vi "Log Reader.vi"() -> ()   [LabVIEW 2012]
uses:
  <vilib>/Utility/sysdir.llb/System Directory Type.ctl
  <vilib>/Utility/inputDevices.llb/closeKeyboard.vi
  <vilib>/Utility/inputDevices.llb/keyboardAcquire.vi
panel:
  in  "Cues":i32[](listbox)
  in  "stop":bool
  out "Total Length":u32
  out "Distance":string
  out "Current Pitch":dbl
  out "AutoTargetPitch":dbl
  out "AutoTargetRotation":dbl
  out "Auto Align":bool
  out "Fine Control Mode":bool
  out "SelectedGoalSubarray":dbl[](array[numeric])
  out "Vision Array":dbl[][](array[numeric])
  in  "-1 Frame":bool
  in  "+1 Frame":bool
  in  "Play Speed":dbl(slide)=1.0 step=0.25 scale=-5.0..5.0
  in  "Play/Pause":bool
  out "Image":T1(plugin-control)
  in  "Step":i32
  out "JS Buttons 3":T2
  out "Joystick 1":cluster{"X":dbl, "Y":dbl}[](graph)
  out "Joystick 2":cluster{"X":dbl, "Y":dbl}[](graph)
  out "JS Buttons 1":T2
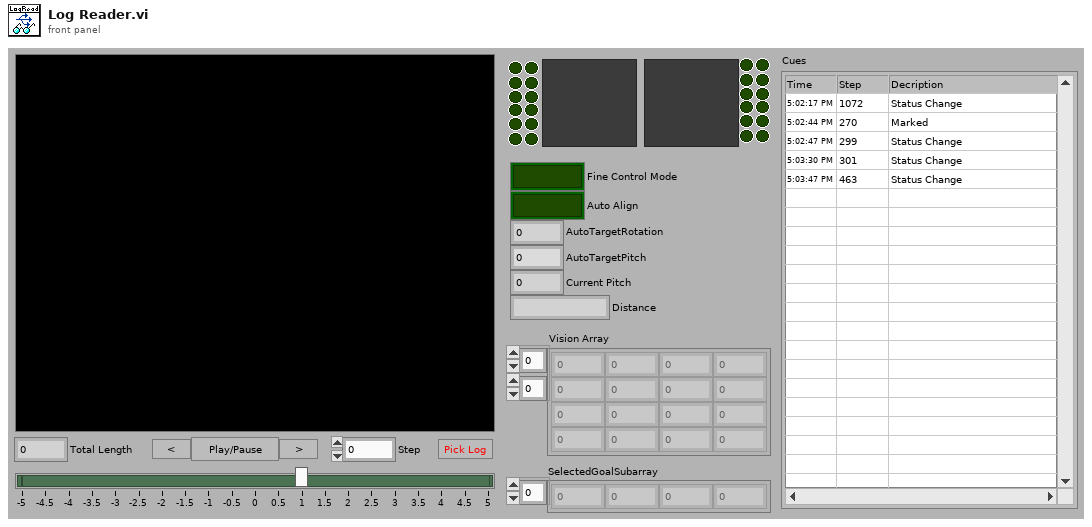
[diagram p1: front panel]
types:
  T1 = typedef "IMAQ Image.ctl" = refnum<image>
  T2 = cluster{bool, bool, bool, bool, bool, bool, bool, bool, bool, bool, bool, bool}
  T3 = cluster{"Joystick 1":cluster{"X":dbl, "Y":dbl}[], "JS Buttons 1":cluster{bool, bool, bool, bool, bool, bool, bool, bool, bool, bool, bool, bool}, "Joystick 2":cluster{"X":dbl, "Y":dbl}[], "JS Buttons 2":cluster{bool, bool, bool, bool, bool, bool, bool, bool, bool, bool, bool, bool}, "AutoTargetRotation":dbl, "AutoTargetPitch":dbl, "Fine Control Mode":bool, "Auto Align":bool, "Current Pitch":dbl, "Full Array":dbl[][], "SelectedGoalSubarray":dbl[], "Distance":string}
  T4 = enum16{"0", "1", "2", "3", "4", "5", "6", "7", "8", "9", "A", "B", "C", "D", "E", "F", "G", "H", "I", "J", "K", "L", "M", "N", "O", "P", "Q", "R", "S", "T", "U", "V", "W", "X", "Y", "Z", "F1", "F2", "F3", "F4", "F5", "F6", "F7", "F8", "F9", "F10", "F11", "F12", "F13", "F14", "F15", "ADD", "BACK", "BACKSLASH", "CAPITAL", "COMMA", "DECIMAL", "DELETE", "DIVIDE", "DOWN", "END", "EQUALS", "ESCAPE", "GRAVE (`)", "HOME", "INSERT", "LBRACKET", "LCONTROL", "LEFT", "L ALT", "LSHIFT", "LWIN", "MINUS", "MULTIPLY", "NEXT", "NUMLOCK", "NUMPAD_0", "NUMPAD_1", "NUMPAD_2", "NUMPAD_3", "NUMPAD_4", "NUMPAD_5", "NUMPAD_6", "NUMPAD_7", "NUMPAD_8", "NUMPAD_9", "PAUSE", "PERIOD", "PRIOR (PG UP)", "RBRACKET", "RCONTROL", "RETURN", "RIGHT", "R ALT", "RSHIFT", "RWIN", "SCROLL", "SEMICOLON", "SLASH", "SPACE", "SUBTRACT", "TAB", "UP", "ENTER (num pad)", "' (quote)"}
  T5 = typedef "System Directory Type.ctl" = i32
  T6 = typedef "Image Type" = u32
  T7 = typedef "AviRefnum.ctl" = refnum<k1>
  T8 = cluster{"Joystick 1":cluster{"X":dbl, "Y":dbl}[], "JS Buttons 1":cluster{bool, bool, bool, bool, bool, bool, bool, bool, bool, bool, bool, bool}, "Joystick 2":cluster{"X":dbl, "Y":dbl}[], "JS Buttons 2":cluster{bool, bool, bool, bool, bool, bool, bool, bool, bool, bool, bool, bool}, "AutoTargetRotation":dbl, "AutoTargetPitch":dbl, "Fine Control Mode":bool, "Auto Align":bool, "Current Pitch":dbl, "Full Array":dbl[][], "SelectedGoalSubarray":dbl[], "Distance":string}[]
  T9 = enum16{"0", "1", "2", "3", "4", "5", "6", "7", "8", "9", "A", "B", "C", "D", "E", "F", "G", "H", "I", "J", "K", "L", "M", "N", "O", "P", "Q", "R", "S", "T", "U", "V", "W", "X", "Y", "Z", "F1", "F2", "F3", "F4", "F5", "F6", "F7", "F8", "F9", "F10", "F11", "F12", "F13", "F14", "F15", "ADD", "BACK", "BACKSLASH", "CAPITAL", "COMMA", "DECIMAL", "DELETE", "DIVIDE", "DOWN", "END", "EQUALS", "ESCAPE", "GRAVE (`)", "HOME", "INSERT", "LBRACKET", "LCONTROL", "LEFT", "L ALT", "LSHIFT", "LWIN", "MINUS", "MULTIPLY", "NEXT", "NUMLOCK", "NUMPAD_0", "NUMPAD_1", "NUMPAD_2", "NUMPAD_3", "NUMPAD_4", "NUMPAD_5", "NUMPAD_6", "NUMPAD_7", "NUMPAD_8", "NUMPAD_9", "PAUSE", "PERIOD", "PRIOR (PG UP)", "RBRACKET", "RCONTROL", "RETURN", "RIGHT", "R ALT", "RSHIFT", "RWIN", "SCROLL", "SEMICOLON", "SLASH", "SPACE", "SUBTRACT", "TAB", "UP", "ENTER (num pad)", "' (quote)"}[]
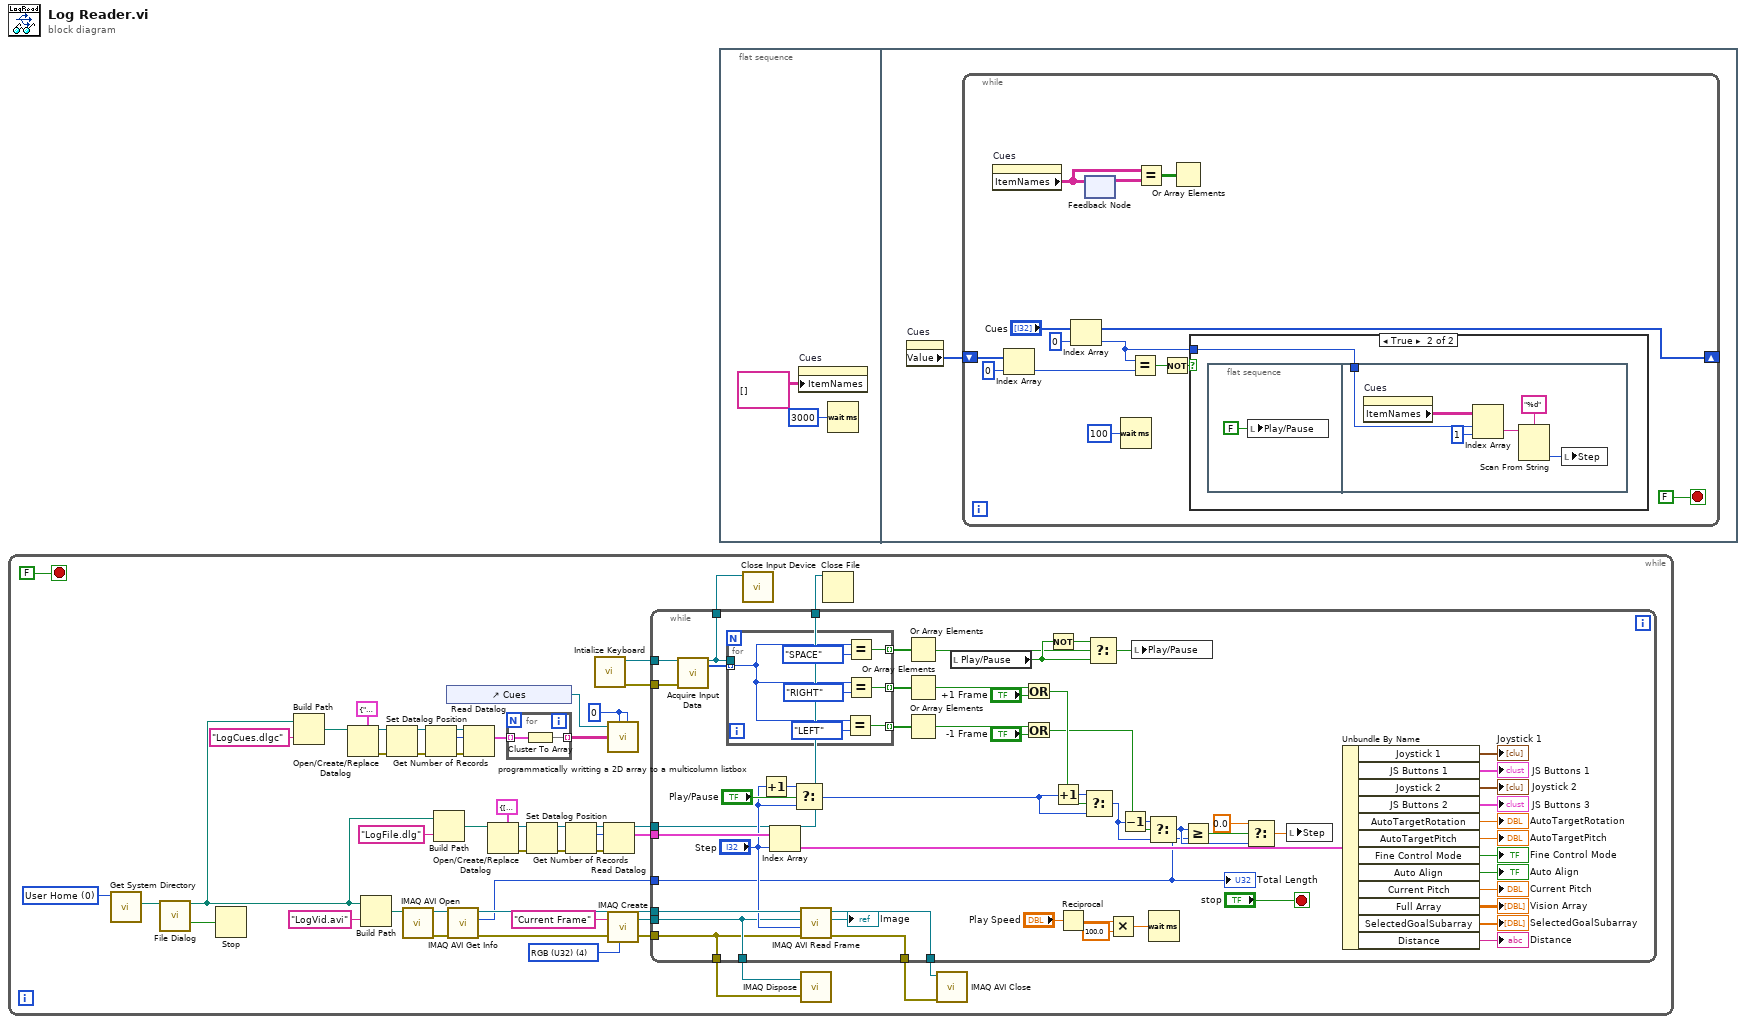
[diagram p0: block diagram]
diagram:
  n1 = while {
    stop <- FALSE stop-if-true
    w2 = 0 ("Start Row")
    w34 = T5 0 items=["User Home"=0, "User Desktop"=1, "User Documents"=2, "User Application Data"=3, "User Preferences"=4, "User Temporary"=5, "Public Documents"=6, "Public Application Data"=7, "Public Preferences"=8, "Public Cache"=13, "System Core Libraries"=9, "System Installed Libraries"=10, "Application Files"=11, "Boot Volume Root"=12] ("system directory type")
    w49 = T6 4 items=["Grayscale (U8)", "Grayscale (I16)", "Grayscale (SGL)", "Complex (CSG)", "RGB (U32)", "HSL (U32)", "RGB (U64)", "Grayscale (U16)"] ("Image Type")
    n2 = call <vilib>:"Get System Directory.vi"("system directory type"=w34) -> ("system directory"=w35:path)  [unwired: 10 in]
    n3 = call "File Dialog"("start path"=w35) -> ("selected path"=w7:path, "cancelled"=w32:bool)  [unwired: 11 in, 2 out]
    n4 = Stop(stop? (T)=w32) -> ()
    n5 = Build Path(base path=w7, name or relative path="LogCues.dlgc") -> (appended path=w8:path)
    n6 = Open/Create/Replace Datalog(5:cluster{string, string, string} {"", "", ""}, 11:w8) -> (0:w10:errorcluster, 3:w6:refnum<k1>)  [unwired: 4 in, 1 out]
    n7 = Build Path(base path=w7, name or relative path="LogVid.avi") -> (appended path=w36:path)
    n8 = Set Datalog Position(4:w10, 7:w6) -> (0:w11:errorcluster, 3:w12:refnum<k1>)  [unwired: 2 in]
    n9 = call "IMAQ AVI Open"("AVI Path"=w36) -> ("error out"=w26:errorcluster, "Avi Refnum"=w31:T7)  [unwired: 9 in]
    n10 = Get Number of Records(4:w11, 7:w12) -> (0:w13:errorcluster, 2:w14:i64, 3:w15:refnum<k1>)
    n11 = Build Path(base path=w7, name or relative path="LogFile.dlg") -> (appended path=w37:path)
    n12 = control-ref of="Cues"() -> (w4:refnum<vi>)
    n13 = call "IMAQ AVI Get Info"("error in (no error)"=w26, "Avi Refnum"=w31) -> ("error out"=w28:errorcluster, "Number of Frames"=w29:u32, "Avi Refnum (duplicate)"=w30:T7)  [unwired: 5 in, 2 out]
    n14 = Read Datalog(4:w13, 6:w14, 7:w15) -> (2:w3:cluster{string, string, string}[])  [unwired: 2 out]
    n15 = Open/Create/Replace Datalog(5:T3 {"Joystick 1"=[], "JS Buttons 1"={FALSE, FALSE, FALSE, FALSE, FALSE, FALSE, FALSE, FALSE, FALSE, FALSE, FALSE, FALSE}, "Joystick 2"=[], "JS Buttons 2"={FALSE, FALSE, FALSE, FALSE, FALSE, FALSE, FALSE, FALSE, FALSE, FALSE, FALSE, FALSE}, "AutoTargetRotation"=0.0, "AutoTargetPitch"=0.0, "Fine Control Mode"=FALSE, "Auto Align"=FALSE, "Current Pitch"=0.0, "Full Array"=[], "SelectedGoalSubarray"=[], "Distance"=""} ("output cluster"), 11:w37) -> (0:w40:errorcluster, 3:w42:refnum<k1>)  [unwired: 4 in, 1 out]
    n16 = for {
      tunnel: w3 -> [w52] mode=indexing
      tunnel: [w51] -> w1 mode=indexing
      n17 = Cluster To Array(cluster=w52) -> (array=w51:string[])
    }
    n18 = Set Datalog Position(4:w40, 7:w42) -> (0:w41:errorcluster, 3:w43:refnum<k1>)  [unwired: 2 in]
    n19 = Get Number of Records(4:w41, 7:w43) -> (0:w44:errorcluster, 2:w45:i64, 3:w46:refnum<k1>)
    n20 = call <vilib>:"Intialize Keyboard.vi"() -> ("error out"=w18:errorcluster, "device ID"=w19:refnum<k1>)  [unwired: 10 in]
    n21 = Read Datalog(4:w44, 6:w45, 7:w46) -> (2:w47:T8, 3:w20:refnum<k1>)  [unwired: 1 out]
    n22 = call "programmatically writting a 2D array to a multicolumn listbox.vi"("MCListbox Refnum"=w4, "Start Row"=w2, "Input 2D Array"=w1, "Start Column"=w2) -> ()  [unwired: 3 in, 3 out]
    n23 = call "IMAQ Create"("Image Name"="Current Frame", "Image Type"=w49, "error in (no error)"=w28) -> ("New Image"=w33:T1, "error out"=w27:errorcluster)  [unwired: 2 in]
    n24 = while {
      tunnel: w47 -> [w106]
      tunnel: w30 -> [w105]
      tunnel: w33 -> [w74]
      tunnel: w29 -> [w81]
      tunnel: w27 -> [w73]
      tunnel: [w74] -> w24
      tunnel: [w73] -> w23
      tunnel: [w72] -> w22
      tunnel: [w71] -> w21
      tunnel: w20 -> [w53]
      tunnel: w19 -> [w70]
      tunnel: w18 -> [w69]
      tunnel: [w54] -> w17
      tunnel: [w53] -> w16
      stop <- "stop" stop-if-true
      n25 = call-poly <vilib>:"Acquire Input Data.vi"("device ID"=w70, "error in (no error)"=w69) -> ("device ID"=w54:refnum<k1>, "keys pressed"=w68:T9)  [unwired: 15 in, 1 out]
      n26 = for {
        tunnel: w68 -> [w114] mode=indexing
        tunnel: w54 -> [_]
        tunnel: [w110] -> w67 mode=indexing
        tunnel: [w109] -> w65 mode=indexing
        tunnel: [w108] -> w66 mode=indexing
        n27 = Equal?(x=w114, y=T4."LEFT") -> (x = y?=w108:bool)
        n28 = Equal?(x=w114, y=T4."SPACE") -> (x = y?=w110:bool)
        n29 = Equal?(x=w114, y=T4."RIGHT") -> (x = y?=w109:bool)
      }
      n30 = Increment(x="Step") -> (x+1=w82:i32)
      n31 = Index Array(array=w106, index="Step") -> (element=w107:T3)
      n32 = Select(t=w82, s="Play/Pause", f="Step") -> (s? t:f=w87:i32)
      n33 = call "IMAQ AVI Read Frame"("error in (no error)"=w73, "Frame Number"="Step", "Image"=w74, "Avi Refnum"=w105) -> ("error out"=w71:errorcluster, "Image Out"=→"Image":T1, "Avi Refnum (duplicate)"=w72:T7)  [unwired: 4 in, 1 out]
      n34 = Or Array Elements(Boolean array=w67) -> (logical OR=w55:bool)
      n35 = Or Array Elements(Boolean array=w65) -> (logical OR=w62:bool)
      n36 = Or Array Elements(Boolean array=w66) -> (logical OR=w63:bool)
      n37 = local read "Play/Pause"() -> (w56:bool)
      n38 = Or(x=w62, y="+1 Frame") -> (x .or. y?=w60:bool)
      n39 = Or(x=w63, y="-1 Frame") -> (x .or. y?=w59:bool)
      n40 = Not(x=w56) -> (.not. x?=w58:bool)
      n41 = Increment(x=w87) -> (x+1=w96:i32)
      n42 = Reciprocal(x="Play Speed") -> (1/x=w79:dbl)
      n43 = Select(t=w96, s=w60, f=w87) -> (s? t:f=w98:i32)
      n44 = Select(t=w58, s=w55, f=w56) -> (s? t:f=w57:bool)
      n45 = Multiply(x=w79, y=100.0) -> (x*y=w76:dbl)
      n46 = Decrement(x=w98) -> (x-1=w97:i32)
      n47 = local write "Play/Pause"(w57) -> ()
      n48 = Select(t=w97, s=w59, f=w98) -> (s? t:f=w83:i32)
      n49 = Wait (ms)(milliseconds to wait=w76) -> ()  [unwired: 1 out]
      n50 = Greater Or Equal?(x=w83, y=w81) -> (x >= y?=w85:bool)
      n51 = Select(t=0.0, s=w85, f=w83) -> (s? t:f=w86:dbl)
      n52 = local write "Step"(w86) -> ()
      n53 = Unbundle By Name(w107) -> ("Joystick 1"=→"Joystick 1":cluster{"X":dbl, "Y":dbl}[], "JS Buttons 1"=→"JS Buttons 1":T2, "Joystick 2"=→"Joystick 2":cluster{"X":dbl, "Y":dbl}[], "JS Buttons 2"=→"JS Buttons 3":T2, "AutoTargetRotation"=→"AutoTargetRotation":dbl, "AutoTargetPitch"=→"AutoTargetPitch":dbl, "Fine Control Mode"=→"Fine Control Mode":bool, "Auto Align"=→"Auto Align":bool, "Current Pitch"=→"Current Pitch":dbl, "Full Array"=→"Vision Array":dbl[][], "SelectedGoalSubarray"=→"SelectedGoalSubarray":dbl[], "Distance"=→"Distance":string)
      "Total Length" <- w81
    }
    n54 = call-poly <vilib>:"Close Input Device.vi"("device ID"=w17) -> ()  [unwired: 9 in, 1 out]
    n55 = call "IMAQ Dispose"("Image"=w24, "error in (no error)"=w23) -> ()  [unwired: 4 in, 1 out]
    n56 = Close File(refnum=w16) -> ()  [unwired: 1 in, 2 out]
    n57 = call "IMAQ AVI Close"("error in (no error)"=w21, "Avi Refnum"=w22) -> ()  [unwired: 9 in, 1 out]
  }
  n58 = flat-sequence {
    frame #0 {
      n59 = property on="Cues" class="MCListbox (strict)"("ItemNames"=string[][] [] ("Item Names")) -> ()  [unwired: 2 in, 2 out]
      n60 = Wait (ms)(milliseconds to wait=u32 3000) -> ()  [unwired: 1 out]
    }
    frame #1 {
      n61 = property on="Cues" class="MCListbox (strict)"() -> ("Value"=w117:i32[])  [unwired: 2 in, 2 out]
      n62 = while {
        shift-right: ["Cues"] -> _
        shift-left: w117 -> [w127]
        stop <- FALSE stop-if-true
        n63 = property on="Cues" class="MCListbox (strict)"() -> ("ItemNames"=w119:string[][])  [unwired: 2 in, 2 out]
        n64 = Index Array(array=w127, index=0) -> (element=w123:i32)
        n65 = Index Array(array="Cues", index=0) -> (element=w122:i32)
        n66 = feedback-in #1(w119) -> ()
        n67 = feedback #1() -> (w120:string[][])  [unwired: 1 in]
        n68 = Wait (ms)(milliseconds to wait=u32 100) -> ()  [unwired: 1 out]
        n69 = Equal?(x=w122, y=w123) -> (x = y?=w129:bool)
        n70 = Equal?(x=w119, y=w120) -> (x = y?=w118:bool[][])
        n71 = Not(x=w129) -> (.not. x?=w128:bool)
        n72 = Or Array Elements(Boolean array=w118) -> ()  [unwired: 1 out]
        n73 = case shown="True" w128 {
          tunnel: w122 -> [_ w131]
          frame False {
          }
          frame True {
            n74 = flat-sequence {
              tunnel: w131 -> [w133]
              frame #0 {
                n75 = local write "Play/Pause"(FALSE ("Play/Pause")) -> ()
              }
              frame #1 {
                n76 = property on="Cues" class="MCListbox (strict)"() -> ("ItemNames"=w138:string[][])  [unwired: 2 in, 2 out]
                n77 = Index Array(array=w138, index (row)=w133, index (col)=1 ("disabled index (col)")) -> (element=w136:string)
                n78 = Scan From String(format string="%d", input string=w136) -> (output 1=w135:i32)  [unwired: 3 in, 3 out]
                n79 = local write "Step"(w135) -> ()
              }
            }
          }
        }
      }
    }
  }
